vi "Disabled And.vi"(1 "Disabled 2":T1(ring), 2 "Disabled 1":T1(ring)) -> (0 "Disabled":T1(ring))   [LabVIEW 2017]
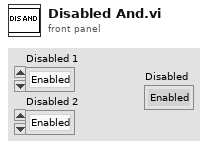
[diagram p1: front panel]
types:
  T1 = enum8{"Enabled", "Disabled", "Disabled and Grayed Out"}
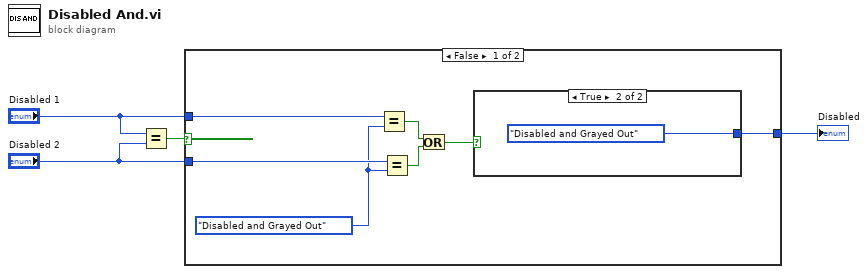
[diagram p0: block diagram]
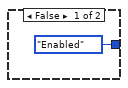
[diagram p2: hidden frame]
diagram:
  n1 = Equal?(x="Disabled 1", y="Disabled 2") -> (x = y?=w4:bool)
  n2 = case shown="False" w4 {
    tunnel: "Disabled 1" -> [w11 _]
    tunnel: "Disabled 2" -> [w10 w14]
    tunnel: [w5 w14] -> w1
    frame False {
      w9 = T1."Disabled and Grayed Out" ("y")
      n3 = Equal?(x=w11, y=w9) -> (x = y?=w7:bool)
      n4 = Equal?(x=w10, y=w9) -> (x = y?=w8:bool)
      n5 = Or(x=w7, y=w8) -> (x .or. y?=w6:bool)
      n6 = case shown="True" w6 {
        tunnel: [T1."Enabled" ("y") T1."Disabled and Grayed Out" ("y")] -> w5
        frame False {
        }
        frame True {
        }
      }
    }
    frame True {
    }
  }
  "Disabled" <- w1
